vi "Relative Accuracy Measurement.vi"(0 "VISA resource name":refnum<visa-resource-name>, 1 "Frequency (20)":dbl=20.0 min=20.0 max=1000000.0 format="%.2f", 5 "Ae Accuracy (0.05)":dbl format="%.3f", 11 "error in (no error)":errorcluster) -> (4 "VISA resource name out":refnum<visa-resource-name>, 6 "Degree Accuracy":dbl format="%^.2e", 8 "Rp Accuracy":dbl format="%^.2e", 10 "Rs Accuracy":dbl format="%^.2e", 12 "D Accuracy":dbl format="%^.2e", 13 "G Accuracy":dbl format="%^.2e", 14 "Q Accuracy":dbl format="%^.2e", 15 "error out":errorcluster)   [LabVIEW 2015, in "Agilent 428X Series.lvlib"]
doc: "This VI is to calculate the relative accuracy of D,G,Theta,Q, Rs,Rp."
uses:
  Agilent 428X Series.lvlib
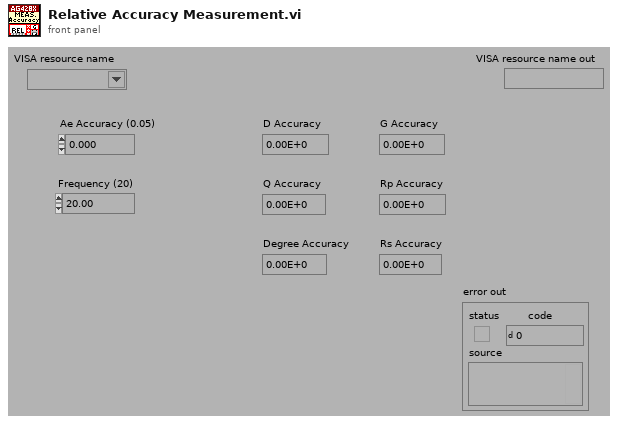
[diagram p1: front panel]
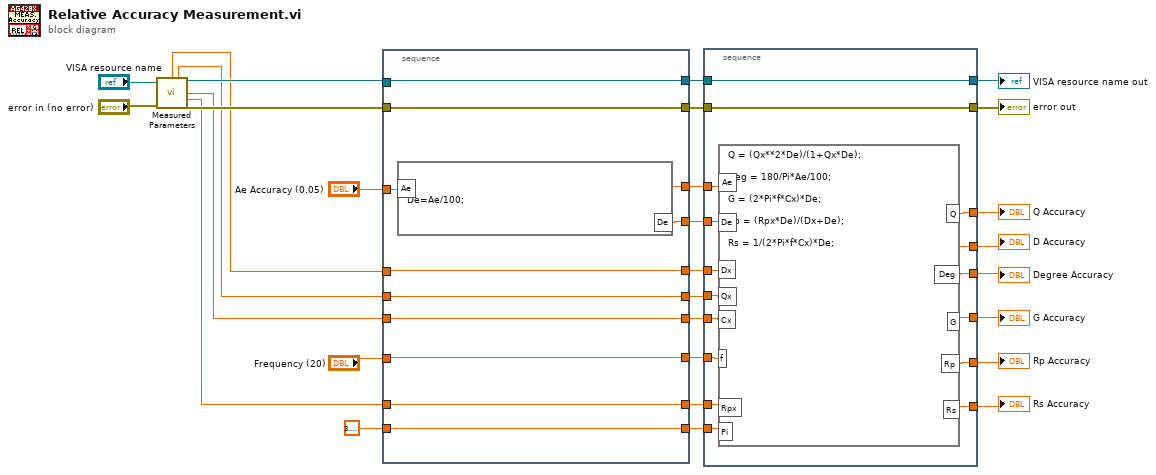
[diagram p0: block diagram]
diagram:
  n1 = call "Measured Parameters.vi"("VISA resource name"="VISA resource name", "error in (no error)"="error in (no error)") -> ("Dx"=w7:dbl, "Qx"=w6:dbl, "VISA resource name out"=w9:refnum<visa-resource-name>, "Cx"=w5:dbl, "Rp"=w4:dbl, "error out"=w8:errorcluster)  [unwired: 7 in, 1 out]
  n2 = stacked-sequence {
    tunnel: w9 -> [w38]
    tunnel: w8 -> [w39]
    tunnel: [w39] -> w18
    tunnel: [w38] -> w20
    tunnel: "Ae Accuracy (0.05)" -> [w37]
    tunnel: [w37] -> w26
    tunnel: [w36] -> w22
    tunnel: w6 -> [w35]
    tunnel: w5 -> [w34]
    tunnel: "Frequency (20)" -> [w33]
    tunnel: w4 -> [w32]
    tunnel: w7 -> [w30]
    tunnel: 3.141592653589793 -> [w31]
    tunnel: [w31] -> w23
    tunnel: [w33] -> w24
    tunnel: [w34] -> w25
    tunnel: [w35] -> w2
    tunnel: [w32] -> w3
    tunnel: [w30] -> w1
    frame #0 {
      n3 = formula code="De=Ae/100;"("Ae"=w37) -> ("De"=w36:dbl)
    }
  }
  n4 = stacked-sequence {
    tunnel: w26 -> [w54]
    tunnel: w2 -> [w53]
    tunnel: w25 -> [w52]
    tunnel: w24 -> [w51]
    tunnel: w3 -> [w50]
    tunnel: w23 -> [w49]
    tunnel: w22 -> [w48]
    tunnel: [w48] -> w21
    tunnel: w20 -> [w47]
    tunnel: [w47] -> w19
    tunnel: w18 -> [w46]
    tunnel: [w46] -> w17
    tunnel: [w45] -> w16
    tunnel: [w44] -> w15
    tunnel: [w43] -> w14
    tunnel: [w42] -> w13
    tunnel: [w41] -> w12
    tunnel: w1 -> [w40]
    frame #0 {
      n5 = formula code="Q = (Qx**2*De)/(1+Qx*De);\n\nDeg = 180/Pi*Ae/100;\n\nG = (2*Pi*f*Cx)*De;\n\nRp = (Rpx*De)/(Dx+De);\n\nRs = 1/(2*Pi*f*Cx)*De;"("Pi"=w49, "Rpx"=w50, "f"=w51, "Cx"=w52, "Qx"=w53, "Dx"=w40, "Ae"=w54, "De"=w48) -> ("Q"=w45:dbl, "Deg"=w44:dbl, "G"=w43:dbl, "Rp"=w42:dbl, "Rs"=w41:dbl)
    }
  }
  "VISA resource name out" <- w19
  "error out" <- w17
  "D Accuracy" <- w21
  "Q Accuracy" <- w16
  "Degree Accuracy" <- w15
  "G Accuracy" <- w14
  "Rp Accuracy" <- w13
  "Rs Accuracy" <- w12
